vi "EnQueue.vi"   [LabVIEW 2013]
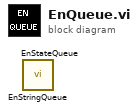
[diagram p0: block diagram]
diagram:
  n1 = call "EnStringQueue.vi"() -> ()  [unwired: 10 in, 2 out]
  n2 = call "EnStateQueue.vi"() -> ()  [unwired: 10 in, 2 out]
